vi "Count Number of Instances in Array.vi"(11 "Input Array":dbl[](array[numeric])) -> (2 "Count":i32[](array[numeric]), 3 "Elements Found":dbl[](array[numeric]))   [LabVIEW 2016]
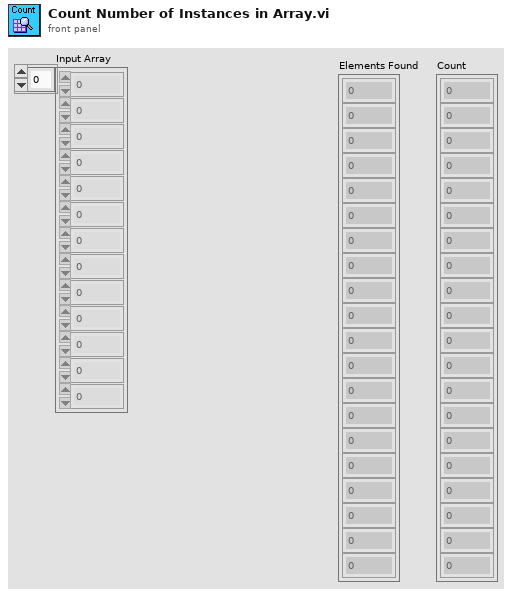
[diagram p1: front panel]
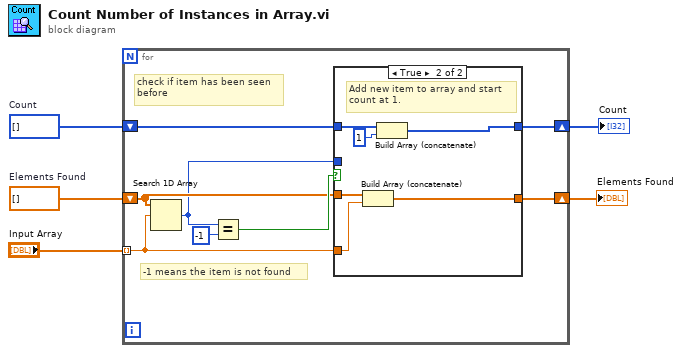
[diagram p0: block diagram]
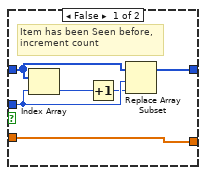
[diagram p2: hidden frame]
diagram:
  w3 = i32[] []  # Count
  w4 = dbl[] []  # Elements Found
  n1 = for {
    tunnel: "Input Array" -> [w10] mode=indexing
    shift-right: [w9] -> w2
    shift-left: w4 -> [w11]
    shift-right: [w7] -> w1
    shift-left: w3 -> [w8]
    # "-1 means the item is not found"
    # "check if item has been seen\nbefore"
    n2 = Search 1D Array(1D array=w11, element=w10) -> (index of element=w6:i32)  [unwired: 1 in]
    n3 = Equal?(x=w6, y=-1) -> (x = y?=w12:bool)
    n4 = case shown="True" w12 {
      tunnel: w11 -> [w19 w25]
      tunnel: w10 -> [_ w24]
      tunnel: [w19 w23] -> w9
      tunnel: w8 -> [w18 w22]
      tunnel: [w14 w20] -> w7
      tunnel: w6 -> [w17 _]
      frame False {
        # "Item has been Seen before,\nincrement count"
        n5 = Index Array(array=w18, index=w17) -> (element=w15:i32)
        n6 = Increment(x=w15) -> (x+1=w16:i32)
        n7 = Replace Array Subset(array=w18, new element=w16, index=w17) -> (w14:i32[])
      }
      frame True {
        # "Add new item to array and start\ncount at 1."
        n8 = Build Array (concatenate)(w25, w24) -> (w23:dbl[])
        n9 = Build Array (concatenate)(w22, 1) -> (w20:i32[])
      }
    }
  }
  "Elements Found" <- w2
  "Count" <- w1
